vi "Array_Investigation.vi"() -> ()   [LabVIEW 2014]
doc: "This VI is an exercise in the LabVIEW Core I course.\n\nEnter the number of columns and rows you want generated, then run the VI. This VI generates an array with the number of rows and columns you specify."
panel:
  out "Second Column":dbl[](array[numeric])
  out "Third Row":dbl[](array[numeric])
  out "Array":dbl[][](array[numeric])
  in  "Rows":i32=80
  in  "Columns":i32=80
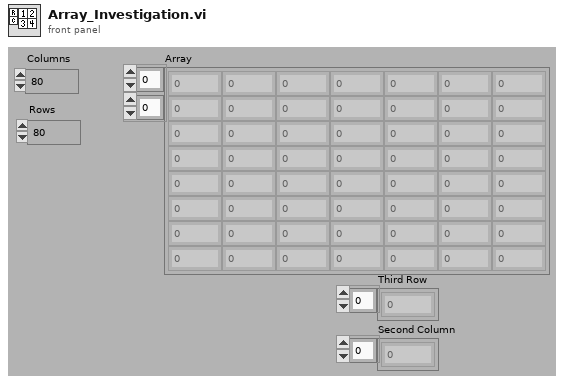
[diagram p1: front panel]
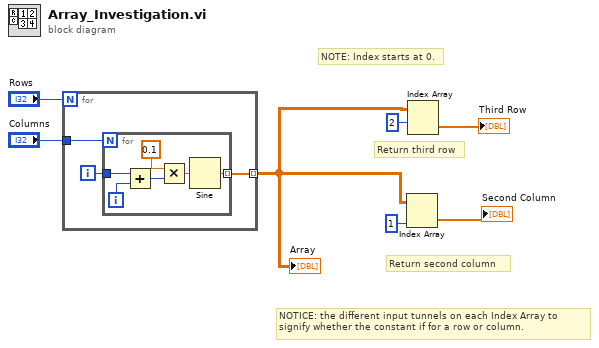
[diagram p0: block diagram]
diagram:
  # "NOTICE: the different input tunnels on each Index Array to \nsignify whether the constant if for a row or column."
  # "NOTE: Index starts at 0."
  # "Return second column"
  # "Return third row"
  n1 = for {
    N: "Rows" -> [_]
    tunnel: [w10] -> w4 mode=indexing
    tunnel: "Columns" -> [w9]
    i -> [w8]
    n2 = for {
      N: w9 -> [_]
      tunnel: [w16] -> w10 mode=indexing
      tunnel: w8 -> [w13]
      i -> [w14]
      n3 = Add(x=w13, y=w14) -> (x+y=w15:i32)
      n4 = Multiply(x=0.1, y=w15) -> (x*y=w12:dbl)
      n5 = Sine(x=w12) -> (sin(x)=w16:dbl)
    }
  }
  "Array" <- w4
  n6 = Index Array(array=w4, index (col)=1 ("disabled index (col)")) -> (element=→"Second Column":dbl[])  [unwired: 1 in]
  n7 = Index Array(array=w4, index (row)=2 ("index")) -> (element=→"Third Row":dbl[])  [unwired: 1 in]
